vi "String Output Item UI Update.vi"(8 "error in (no error)":errorcluster, 10 "String UI Elements":T1, 11 "Output":T2) -> (0 "error out":errorcluster)   [LabVIEW 2015, in "OutputUI.lvclass"]
uses:
  OutputUI.lvclass
  Step/STEP_OUTPUT.ctl
  Step/OUTPUT_DATA_TYPE.ctl
  OUTPUT_CHECK_TYPE.ctl
  Step/OUTPUT_VALUE_TYPE.ctl
  Step.lvclass
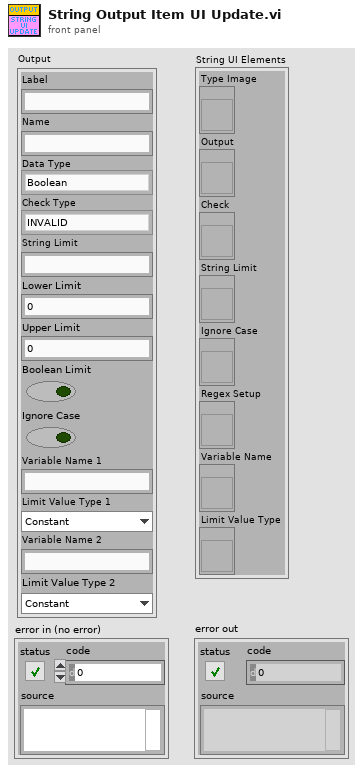
[diagram p1: front panel]
types:
  T1 = cluster{"Type Image":refnum<vi>, "Output":refnum<vi>, "Check":refnum<vi>, "String Limit":refnum<vi>, "Ignore Case":refnum<vi>, "Regex Setup":refnum<vi>, "Variable Name":refnum<vi>, "Limit Value Type":refnum<vi>}
  T2 = typedef "Step.lvclass/STEP_OUTPUT.ctl" = cluster{"Label":string, "Name":string, "Data Type":T3, "Check Type":T4, "String Limit":string, "Lower Limit":dbl, "Upper Limit":dbl, "Boolean Limit":bool, "Ignore Case":bool, "Variable Name 1":string, "Limit Value Type 1":T5, "Variable Name 2":string, "Limit Value Type 2":T5}
  T3 = typedef "Step.lvclass/OUTPUT_DATA_TYPE.ctl" = enum16{"Boolean", "String", "Numeric", "Other"}
  T4 = typedef "Step.lvclass/OUTPUT_CHECK_TYPE.ctl" = enum16{"INVALID", "DO_NOT_CHECK", "RECORD", "VARIABLE", "EQUAL", "NOT_EQUAL", "STR_CONTAINS", "STR_START_WITH", "STR_END_WITH", "STR_REGEX_MATCH", "NUM_GT", "NUM_LT", "NUM_GE", "NUM_LE", "NUM_RANGE", "NUM_RANGE_BDY"}
  T5 = typedef "Step.lvclass/OUTPUT_VALUE_TYPE.ctl" = enum16{"Constant", "Variable"}
  T6 = enum8{"Enabled", "Disabled", "Disabled and Grayed Out"}
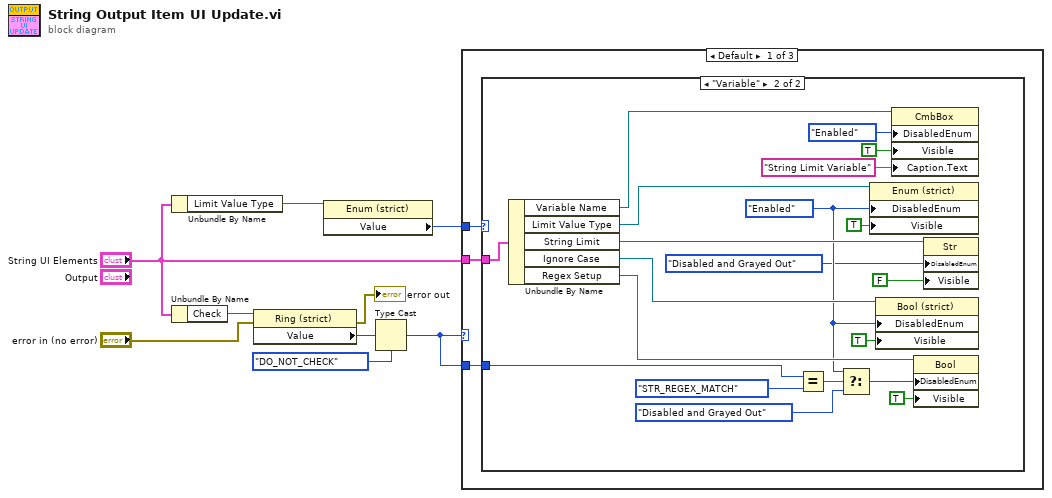
[diagram p0: block diagram]
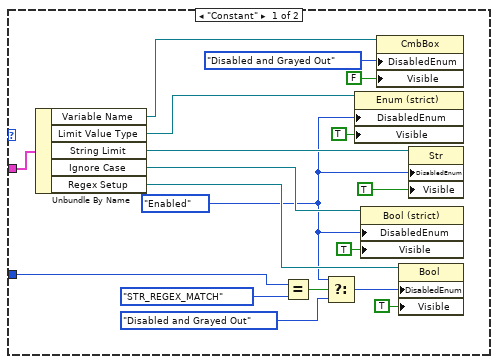
[diagram p2: hidden frame]
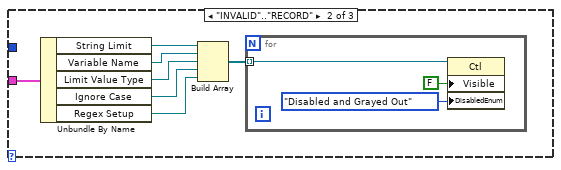
[diagram p3: hidden frame]
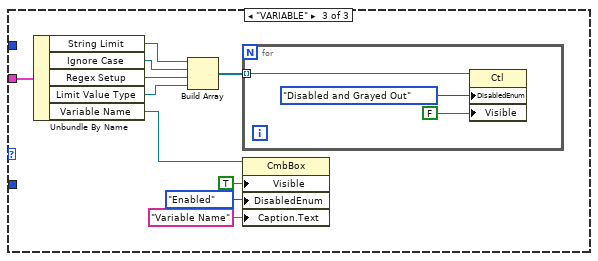
[diagram p4: hidden frame]
diagram:
  n1 = Unbundle By Name("String UI Elements") -> ("Limit Value Type"=w3:refnum<vi>)
  n2 = Unbundle By Name("String UI Elements") -> ("Check"=w9:refnum<vi>)
  n3 = property class="Ring (strict)"(reference=w9, error in="error in (no error)") -> (error out=→"error out":errorcluster, "Value"=w7:u16)  [unwired: 1 out]
  n4 = property class="Enum (strict)"(reference=w3) -> ("Value"=w2:T5)  [unwired: 1 in, 2 out]
  n5 = Type Cast(type=OUTPUT_CHECK_TYPE."DO_NOT_CHECK" ("Check Type"), x=w7) -> (*(type *) &x=w5:T4)
  n6 = case shown="Default" w5 {
    tunnel: "String UI Elements" -> [w12 w53 w70]
    tunnel: w2 -> [w11 _ _]
    tunnel: w5 -> [w10 _ _]
    frame Default {
      n7 = case shown="\"Variable\"" w11 {
        tunnel: w12 -> [w23 w43]
        tunnel: w10 -> [w22 w42]
        frame "Constant" {
          w15 = T6."Enabled" ("Disabled")
          n8 = Unbundle By Name(w23) -> ("Variable Name"=w18:refnum<vi>, "Limit Value Type"=w16:refnum<vi>, "String Limit"=w24:refnum<vi>, "Ignore Case"=w25:refnum<vi>, "Regex Setup"=w26:refnum<vi>)
          n9 = Equal?(x=w22, y=OUTPUT_CHECK_TYPE."STR_REGEX_MATCH" ("Check Type")) -> (x = y?=w28:bool)
          n10 = Select(t=w15, s=w28, f=T6."Disabled and Grayed Out") -> (s? t:f=w29:T6)
          n11 = property class="Enum (strict)"(reference=w16, "DisabledEnum"=w15, "Visible"=TRUE) -> ()  [unwired: 1 in, 2 out]
          n12 = property class="Bool (strict)"(reference=w25, "DisabledEnum"=w15, "Visible"=TRUE) -> ()  [unwired: 1 in, 2 out]
          n13 = property class="CmbBox"(reference=w18, "DisabledEnum"=T6."Disabled and Grayed Out" ("Disabled"), "Visible"=FALSE) -> ()  [unwired: 1 in, 2 out]
          n14 = property class="Bool"(reference=w26, "DisabledEnum"=w29, "Visible"=TRUE) -> ()  [unwired: 1 in, 2 out]
          n15 = property class="Str"(reference=w24, "DisabledEnum"=w15, "Visible"=TRUE) -> ()  [unwired: 1 in, 2 out]
        }
        frame "Variable" {
          w32 = T6."Enabled" ("Disabled")
          n16 = Unbundle By Name(w43) -> ("Variable Name"=w38:refnum<vi>, "Limit Value Type"=w36:refnum<vi>, "String Limit"=w44:refnum<vi>, "Ignore Case"=w45:refnum<vi>, "Regex Setup"=w46:refnum<vi>)
          n17 = Equal?(x=w42, y=OUTPUT_CHECK_TYPE."STR_REGEX_MATCH" ("Check Type")) -> (x = y?=w48:bool)
          n18 = Select(t=w32, s=w48, f=T6."Disabled and Grayed Out") -> (s? t:f=w49:T6)
          n19 = property class="Enum (strict)"(reference=w36, "DisabledEnum"=w32, "Visible"=TRUE) -> ()  [unwired: 1 in, 2 out]
          n20 = property class="Bool (strict)"(reference=w45, "DisabledEnum"=w32, "Visible"=TRUE) -> ()  [unwired: 1 in, 2 out]
          n21 = property class="CmbBox"(reference=w38, "DisabledEnum"=T6."Enabled" ("Disabled"), "Visible"=TRUE, "Caption.Text"="String Limit Variable" ("format string")) -> ()  [unwired: 1 in, 2 out]
          n22 = property class="Bool"(reference=w46, "DisabledEnum"=w49, "Visible"=TRUE) -> ()  [unwired: 1 in, 2 out]
          n23 = property class="Str"(reference=w44, "DisabledEnum"=T6."Disabled and Grayed Out" ("Disabled"), "Visible"=FALSE) -> ()  [unwired: 1 in, 2 out]
        }
      }
    }
    frame "INVALID".."RECORD" {
      n24 = Unbundle By Name(w53) -> ("String Limit"=w57:refnum<vi>, "Variable Name"=w56:refnum<vi>, "Limit Value Type"=w55:refnum<vi>, "Ignore Case"=w52:refnum<vi>, "Regex Setup"=w51:refnum<vi>)
      n25 = Build Array(w57, w56, w55, w52, w51) -> (w54:refnum<vi>[])
      n26 = for {
        tunnel: w54 -> [w60] mode=indexing
        n27 = property class="Ctl"(reference=w60, "Visible"=FALSE, "DisabledEnum"=T6."Disabled and Grayed Out" ("Disabled")) -> ()  [unwired: 1 in, 2 out]
      }
    }
    frame "VARIABLE" {
      n28 = Unbundle By Name(w70) -> ("String Limit"=w61:refnum<vi>, "Ignore Case"=w62:refnum<vi>, "Regex Setup"=w69:refnum<vi>, "Limit Value Type"=w68:refnum<vi>, "Variable Name"=w64:refnum<vi>)
      n29 = Build Array(w61, w62, w69, w68) -> (w67:refnum<vi>[])
      n30 = for {
        tunnel: w67 -> [w73] mode=indexing
        n31 = property class="Ctl"(reference=w73, "DisabledEnum"=T6."Disabled and Grayed Out" ("Disabled"), "Visible"=FALSE) -> ()  [unwired: 1 in, 2 out]
      }
      n32 = property class="CmbBox"(reference=w64, "Visible"=TRUE, "DisabledEnum"=T6."Enabled" ("Disabled"), "Caption.Text"="Variable Name" ("format string")) -> ()  [unwired: 1 in, 2 out]
    }
  }
